vi "Config Aout Bounds.vi"(6 "Lower Loss (-10.0 V)":dbl=-10.0 min=-160.0 max=160.0 format="%#_6f", 7 "Upper Capacitance (10.0 V)":dbl=10.0 min=-160.0 max=160.0 format="%#_6f", 8 "error in":errorcluster, 9 "Lower Capacitance (-10.0 V)":dbl=-10.0 min=-160.0 max=160.0 format="%#_6f", 10 "Upper Loss (10.0 V)":dbl=10.0 min=-160.0 max=160.0 format="%#_6f", 11 "VISA resource name":refnum<visa-resource-name>) -> (0 "error out":errorcluster, 3 "VISA resource name out":refnum<visa-resource-name>)   [LabVIEW 2018, in "Andeen-Hagerling 2700.lvlib"]
doc: "This VI sets the upper and lower bounds of the capacitance and loss channel output voltages in volts. These output voltage bounds correspond directly to the upper and lower bounds of the deviation capacitance and loss spans in pF and jpF respectively."
uses:
  Andeen-Hagerling 2700.lvlib
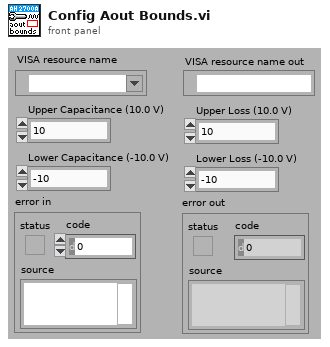
[diagram p1: front panel]
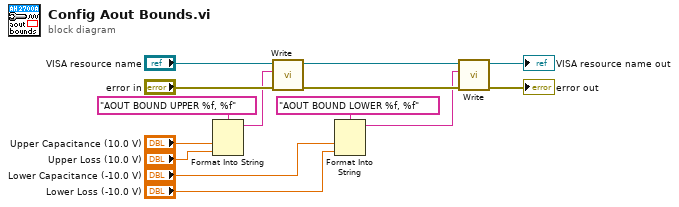
[diagram p0: block diagram]
diagram:
  n1 = Format Into String(format string="AOUT BOUND UPPER %f, %f", "Upper Capacitance (10.0 V)", "Upper Loss (10.0 V)") -> (resulting string=w9:string)  [unwired: 2 in, 1 out]
  n2 = call "Write.vi"("error in"="error in", "command"=w9, "VISA resource name"="VISA resource name") -> ("error out"=w6:errorcluster, "VISA resource name out"=w8:refnum<visa-resource-name>)  [unwired: 7 in]
  n3 = Format Into String(format string="AOUT BOUND LOWER %f, %f", "Lower Capacitance (-10.0 V)", "Lower Loss (-10.0 V)") -> (resulting string=w2:string)  [unwired: 2 in, 1 out]
  n4 = call "Write.vi"("error in"=w6, "command"=w2, "VISA resource name"=w8) -> ("error out"=→"error out":errorcluster, "VISA resource name out"=→"VISA resource name out":refnum<visa-resource-name>)  [unwired: 7 in]
